vi "Get Digest.vi"(11 "Hash Function in":refnum<class "NI_SHA-3.lvclass">) -> (2 "digest":u8[](array[numeric]) format="%02x", 3 "Hash Function out":refnum<class "NI_SHA-3.lvclass">)   [LabVIEW 2020, in "NI_SHA-3.lvclass"]
doc: "Compute the message digest given previously supplied input blocks."
uses:
  <vilib>/security/Message Digest/SHA-3/NI_SHA-3.lvclass
  <vilib>/security/Message Digest/SHA-3/NI_SHA-3.lvclass/NI_SHA-3.ctl
  31857afe-6677-4a2f-85a8-d2efd4cc115e.vi
  31857afe-6677-4a2f-85a8-d2efd4cc115e.vi/a5a20b03-5cce-4b9f-9f05-caa456c51e3e.vi
  31857afe-6677-4a2f-85a8-d2efd4cc115e.vi/97449588-05e4-3fdc-5462-85b544f9ef3f.vi
  <vilib>/security/Message Digest/SHA-3/subVIs/Get State.vi
  31857afe-6677-4a2f-85a8-d2efd4cc115e.vi/504ca6d8-6afe-448d-af66-f2c5cbb3f55e.vi
  <vilib>/security/Message Digest/SHA-3/subVIs/Get Capacity.vi
  31857afe-6677-4a2f-85a8-d2efd4cc115e.vi/97449588-05e4-3fdc-5462-85b544f9ef3f.vi/a7ca2ffa-5243-3fe6-20ad-62a44a00a03f.vi
  31857afe-6677-4a2f-85a8-d2efd4cc115e.vi/97449588-05e4-3fdc-5462-85b544f9ef3f.vi/56df95e4-00ed-3fe6-63c7-84387990dd3f.vi
  31857afe-6677-4a2f-85a8-d2efd4cc115e.vi/97449588-05e4-3fdc-5462-85b544f9ef3f.vi/15d463f4-83a4-3fe1-60d2-4df4fb80bb3f.vi
  31857afe-6677-4a2f-85a8-d2efd4cc115e.vi/97449588-05e4-3fdc-5462-85b544f9ef3f.vi/00016c94-ce57-3fd5-80ac-6e43aea4d93f.vi
  31857afe-6677-4a2f-85a8-d2efd4cc115e.vi/97449588-05e4-3fdc-5462-85b544f9ef3f.vi/7d6bddb0-77c0-3fef-1a90-2ad371c4e73f.vi
  31857afe-6677-4a2f-85a8-d2efd4cc115e.vi/97449588-05e4-3fdc-5462-85b544f9ef3f.vi/fc4e4f9c-ad6e-3fe1-d0d3-ace572eac73f.vi
  31857afe-6677-4a2f-85a8-d2efd4cc115e.vi/97449588-05e4-3fdc-5462-85b544f9ef3f.vi/8eeedd20-ad32-3fe2-c05e-9804496fc23f.vi
  31857afe-6677-4a2f-85a8-d2efd4cc115e.vi/97449588-05e4-3fdc-5462-85b544f9ef3f.vi/cdb60cbe-b6ce-3fe5-5858-44161e95e03f.vi
  31857afe-6677-4a2f-85a8-d2efd4cc115e.vi/97449588-05e4-3fdc-5462-85b544f9ef3f.vi/42a622f8-f126-3fd2-ded5-5715bf86e43f.vi
  31857afe-6677-4a2f-85a8-d2efd4cc115e.vi/97449588-05e4-3fdc-5462-85b544f9ef3f.vi/c2510adc-9471-3fe0-ec8d-87d28ce6de3f.vi
  31857afe-6677-4a2f-85a8-d2efd4cc115e.vi/97449588-05e4-3fdc-5462-85b544f9ef3f.vi/d91c4ef8-a10c-3fd3-c8a5-ddaf779bdf3f.vi
  31857afe-6677-4a2f-85a8-d2efd4cc115e.vi/97449588-05e4-3fdc-5462-85b544f9ef3f.vi/5ec7145c-0dbe-3fe5-90d5-bb6f3223d13f.vi
  31857afe-6677-4a2f-85a8-d2efd4cc115e.vi/97449588-05e4-3fdc-5462-85b544f9ef3f.vi/75751900-1e38-3f99-50ee-d5dc298ed93f.vi
  31857afe-6677-4a2f-85a8-d2efd4cc115e.vi/97449588-05e4-3fdc-5462-85b544f9ef3f.vi/3d4c2402-5c82-3fee-8093-3d672564ba3f.vi
  31857afe-6677-4a2f-85a8-d2efd4cc115e.vi/97449588-05e4-3fdc-5462-85b544f9ef3f.vi/25b0cbf0-9206-3fe6-e0f9-9b2bf19cba3f.vi
  31857afe-6677-4a2f-85a8-d2efd4cc115e.vi/97449588-05e4-3fdc-5462-85b544f9ef3f.vi/f9693195-f45f-3fed-20e0-3dc5325ad03f.vi
  31857afe-6677-4a2f-85a8-d2efd4cc115e.vi/97449588-05e4-3fdc-5462-85b544f9ef3f.vi/3c39b38f-8da6-3fea-2c1c-d149f695dd3f.vi
  31857afe-6677-4a2f-85a8-d2efd4cc115e.vi/97449588-05e4-3fdc-5462-85b544f9ef3f.vi/d15b5a2c-b876-3fe5-7c80-fbd26a60ea3f.vi
  31857afe-6677-4a2f-85a8-d2efd4cc115e.vi/97449588-05e4-3fdc-5462-85b544f9ef3f.vi/bbd71a6c-bf22-3fd6-e4c0-87be6f0be63f.vi
  31857afe-6677-4a2f-85a8-d2efd4cc115e.vi/97449588-05e4-3fdc-5462-85b544f9ef3f.vi/8ddbc49c-000e-3fe3-d243-b9745f7ce73f.vi
  31857afe-6677-4a2f-85a8-d2efd4cc115e.vi/97449588-05e4-3fdc-5462-85b544f9ef3f.vi/b9fabce2-7762-3fee-a034-bf80f1f1ef3f.vi
  31857afe-6677-4a2f-85a8-d2efd4cc115e.vi/504ca6d8-6afe-448d-af66-f2c5cbb3f55e.vi/adab753b-74c4-4997-bc42-33b2ccf3ae86.vi
  <vilib>/security/Message Digest/SHA-3/subVIs/Get Word Type.vi
  <vilib>/security/Message Digest/SHA-3/subVIs/All Rounds.vi
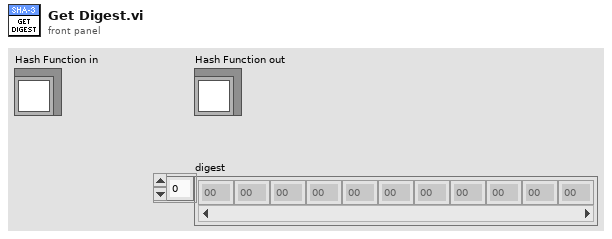
[diagram p1: front panel]
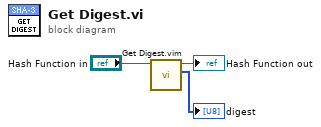
[diagram p0: block diagram]
diagram:
  n1 = call "Get Digest.vim"("Hash Function in"="Hash Function in") -> ("digest"=→"digest":u8[], "Hash Function out"=→"Hash Function out":refnum<class "NI_SHA-3.lvclass">)  [unwired: 9 in]
